vi "Stop FVG.vi"(6 "Stop if error (T)":bool=TRUE, 7 "Akcja (GET)":T1, 8 "Stop in (F)":bool, 11 "error in (no error)":errorcluster) -> (0 "Stop out":bool, 3 "error out":errorcluster)   [LabVIEW 2014]
doc: "Use this template to build a VI to use as a subVI."
uses:
  Kontrolki/FVGs/FVG akcje podstawowa.ctl
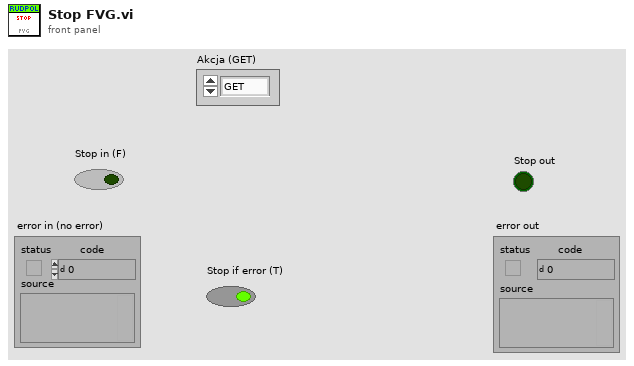
[diagram p1: front panel]
types:
  T1 = typedef "FVG akcje podstawowa.ctl" = enum16{"GET", "SET"}
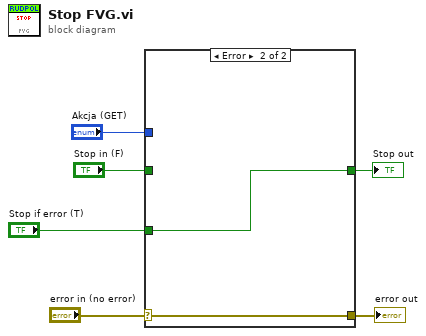
[diagram p0: block diagram]
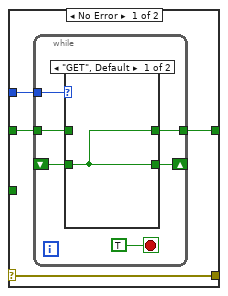
[diagram p2: hidden frame]
diagram:
  n1 = case shown="Error" "error in (no error)" {
    selector: "error in (no error)" -> [w10 w20]
    tunnel: [w10 w20] -> w5
    tunnel: "Stop in (F)" -> [w9 _]
    tunnel: [w8 w19] -> w3
    tunnel: "Akcja (GET)" -> [w7 _]
    tunnel: "Stop if error (T)" -> [_ w19]
    frame No Error {
      n2 = while {
        tunnel: w9 -> [w16]
        shift-right: [w14] -> _
        shift-left: _ -> [w12]
        tunnel: [w13] -> w8
        tunnel: w7 -> [w11]
        stop <- TRUE stop-if-true
        n3 = case shown="\"GET\", Default" w11 {
          tunnel: w16 -> [_ w18]
          tunnel: [w17 w18] -> w14
          tunnel: [w17 w18] -> w13
          tunnel: w12 -> [w17 _]
          frame "GET", Default {
          }
          frame "SET" {
          }
        }
      }
    }
    frame Error {
    }
  }
  "error out" <- w5
  "Stop out" <- w3
